vi "Write Sudoku String.vi"(8 "error in (no error)":errorcluster, 10 "Sudoku String":T1, 11 "Sudoku Class in":refnum<class "Sudoku Class.lvclass">) -> (0 "error out":errorcluster, 3 "Sudoku Class out":refnum<class "Sudoku Class.lvclass">)   [LabVIEW 2015, in "Sudoku Library.lvlib" / "Sudoku Class.lvclass"]
uses:
  Sudoku Class.lvclass
  TypeDef/Sudoku String.ctl
  Sudoku Class.lvclass/Sudoku Class.ctl
  Sudoku Library.lvlib
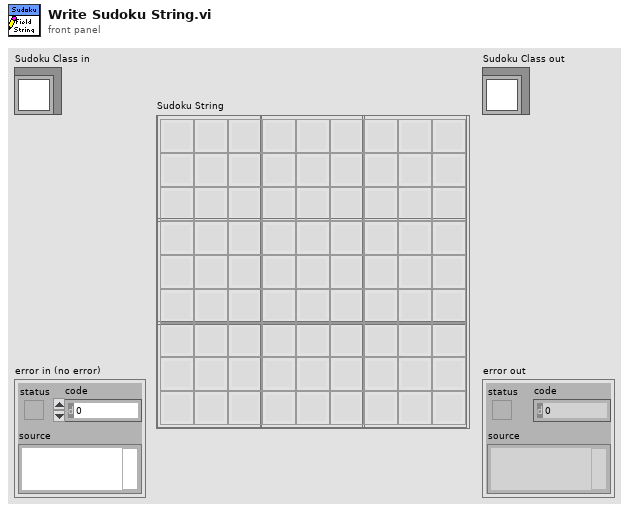
[diagram p1: front panel]
types:
  T1 = typedef "Sudoku Library.lvlib/Sudoku String.ctl" = string[][]
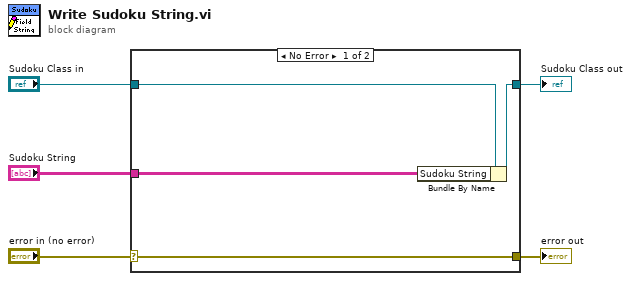
[diagram p0: block diagram]
diagram:
  n1 = case shown="No Error" "error in (no error)" {
    selector: "error in (no error)" -> [w9 w10]
    tunnel: [w9 w10] -> w4
    tunnel: [w7 w11] -> w2
    tunnel: "Sudoku Class in" -> [w8 w11]
    tunnel: "Sudoku String" -> [w6 _]
    frame No Error {
      n2 = Bundle By Name(cluster=w8, "Sudoku String"=w6) -> (w7:refnum<class "Sudoku Class.lvclass">)
    }
    frame Error {
    }
  }
  "error out" <- w4
  "Sudoku Class out" <- w2
